vi "set_wl.vi"(7 "milliseconds to wait":u32=300, 8 "error in (no error)":errorcluster, 10 "fundamental (nm)":dbl=644.431, 11 "VISA resource name":refnum<visa-resource-name>="COM9") -> (0 "error out":errorcluster, 2 "write buffer":string="SL 645.20000000\r\n", 3 "VISA resource name out":refnum<visa-resource-name>="COM9")   [LabVIEW 2017, in "radiant.lvlib"]
doc: "<B>Laser Goto with FCU</B> VI tunes laser to the position <B>Wavenumber (1/cm)</B>. FCU1 is adjusted accordingly."
uses:
  <vilib>/Instr/_visa.llb/VISA Configure Serial Port (Instr).vi
  radiant.lvlib
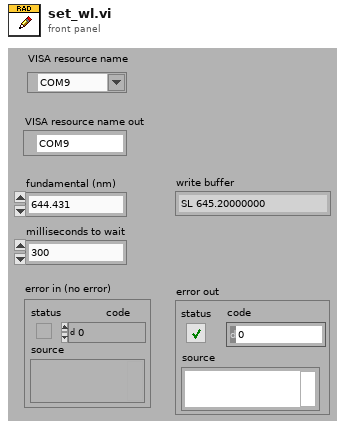
[diagram p1: front panel]
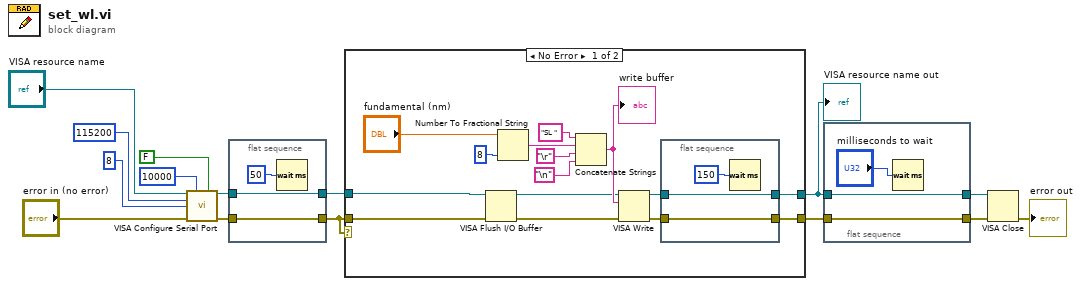
[diagram p0: block diagram]
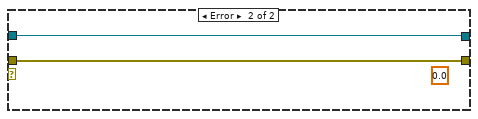
[diagram p2: hidden frame]
diagram:
  n1 = call-poly "VISA Configure Serial Port"("VISA resource name"="VISA resource name", "timeout (10sec)"=u32 10000, "Enable Termination\nChar (T)"=FALSE ("Enable Termination\nChar (T)"), "baud rate (9600)"=u32 115200, "data bits (8)"=u16 8, "error in (no error)"="error in (no error)") -> ("VISA resource name out"=w8:refnum<visa-resource-name>, "error out"=w6:errorcluster)  [unwired: 8 in]
  n2 = flat-sequence {
    tunnel: w8 -> [w18]
    tunnel: [w18] -> w7
    tunnel: w6 -> [w17]
    tunnel: [w17] -> w5
    frame #0 {
      n3 = Wait (ms)(milliseconds to wait=u32 50) -> ()  [unwired: 1 out]
    }
  }
  n4 = case shown="No Error" w5 {
    tunnel: w5 -> [w30 w38]
    tunnel: w7 -> [w29 w37]
    tunnel: [w20 w38] -> w3
    tunnel: [w19 w37] -> w4
    frame No Error {
      n5 = VISA Flush I/O Buffer(VISA resource name=w29, error in (no error)=w30) -> (VISA resource name out=w28:refnum<visa-resource-name>, error out=w27:errorcluster)  [unwired: 1 in]
      n6 = Number To Fractional String(number="fundamental (nm)", precision (6)=i16 8) -> (F-format string=w21:string)  [unwired: 2 in]
      n7 = Concatenate Strings("SL " ("write"), w21, "\r", "\n") -> (w31:string)
      "write buffer" <- w31
      n8 = VISA Write(VISA resource name=w28, write buffer=w31, error in (no error)=w27) -> (VISA resource name out=w26:refnum<visa-resource-name>, error out=w25:errorcluster)  [unwired: 1 out]
      n9 = flat-sequence {
        tunnel: w26 -> [w36]
        tunnel: [w36] -> w19
        tunnel: w25 -> [w35]
        tunnel: [w35] -> w20
        frame #0 {
          n10 = Wait (ms)(milliseconds to wait=u32 150) -> ()  [unwired: 1 out]
        }
      }
    }
    frame Error {
      (unwired) 0.0
    }
  }
  "VISA resource name out" <- w4
  n11 = flat-sequence {
    tunnel: w4 -> [w41]
    tunnel: [w41] -> w1
    tunnel: w3 -> [w40]
    tunnel: [w40] -> w2
    frame #0 {
      n12 = Wait (ms)(milliseconds to wait="milliseconds to wait") -> ()  [unwired: 1 out]
    }
  }
  n13 = VISA Close(VISA resource name=w1, error in (no error)=w2) -> (error out=→"error out":errorcluster)
